vi "read_http_timeout.vi"(8 "error in (no error)":errorcluster, 11 "config_file_name":string) -> (0 "error out":errorcluster, 2 "values":cluster{"get_timeout":i32, "post_timeout":i32}, 3 "config_file_name_out":string)   [LabVIEW 2015]
uses:
  <vilib>/Utility/config.llb/Read Key (String).vi
  <vilib>/Utility/config.llb/NI_LVConfig.lvlib
panel:
  # "Devuelve datos de la sección TIMEOUT del archivo de configuración"
  # "in miliseconds"
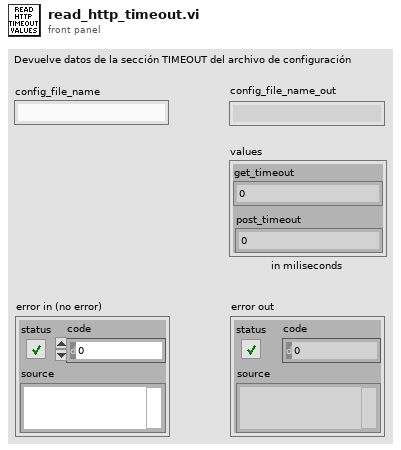
[diagram p1: front panel]
types:
  T1 = typedef "NI_LVConfig.lvlib/Config Data RefNum.ctl" = refnum<k1>
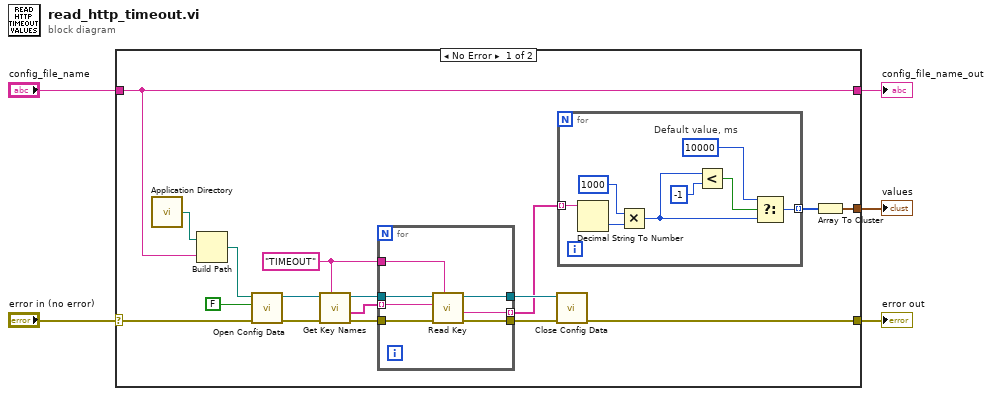
[diagram p0: block diagram]
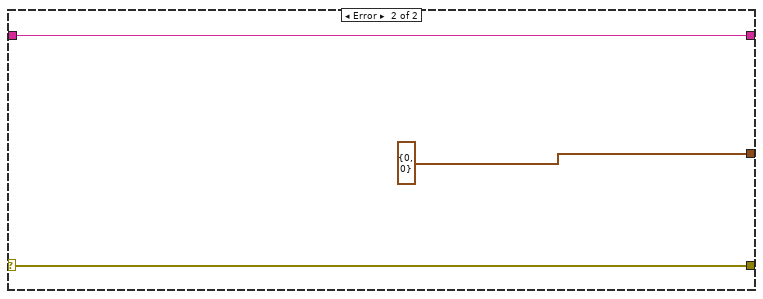
[diagram p2: hidden frame]
diagram:
  n1 = case shown="No Error" "error in (no error)" {
    selector: "error in (no error)" -> [w13 w40]
    tunnel: [w12 w40] -> w5
    tunnel: [w11 w39] -> w3
    tunnel: "config_file_name" -> [w11 w39]
    tunnel: [w8 cluster{"[0]":i32, "[1]":i32} {"[0]"=0, "[1]"=0}] -> w1
    frame No Error {
      w18 = "TIMEOUT" ("section")
      n2 = call <vilib>:"Application Directory.vi"() -> ("Application Directory"=w20:path)
      n3 = Build Path(base path=w20, name or relative path=w11) -> (appended path=w19:path)
      n4 = call <vilib>:"Open Config Data.vi"("error in (no error)"=w13, "create file if necessary (T)"=FALSE, "configuration file path"=w19) -> ("error out"=w22:errorcluster, "refnum"=w21:T1)  [unwired: 6 in, 1 out]
      n5 = call <vilib>:"Get Key Names.vi"("section"=w18, "error in (no error)"=w22, "refnum"=w21) -> ("error out"=w16:errorcluster, "key names"=w10:string[], "refnum out"=w17:T1)  [unwired: 5 in, 1 out]
      n6 = for {
        tunnel: w10 -> [w37] mode=indexing
        tunnel: [w36] -> w7 mode=indexing
        tunnel: w18 -> [w35]
        tunnel: w17 -> [w34]
        tunnel: w16 -> [w33]
        tunnel: [w32] -> w15
        tunnel: [w31] -> w14
        n7 = call-poly <vilib>:"Read Key.vi"("section"=w35, "error in (no error)"=w33, "key"=w37, "refnum"=w34) -> ("error out"=w31:errorcluster, "value"=w36:string, "refnum out"=w32:T1)  [unwired: 4 in, 1 out]
      }
      n8 = call <vilib>:"Close Config Data.vi"("error in (no error)"=w14, "refnum"=w15) -> ("error out"=w12:errorcluster)  [unwired: 8 in, 1 out]
      n9 = for {
        tunnel: w7 -> [w30] mode=indexing
        tunnel: [w27] -> w6 mode=indexing
        # "Default value, ms"
        n10 = Decimal String To Number(string=w30) -> (number=w29:i32)  [unwired: 2 in, 1 out]
        n11 = Multiply(x=1000, y=w29) -> (x*y=w23:i32)
        n12 = Less?(x=w23, y=-1) -> (x < y?=w24:bool)
        n13 = Select(t=10000, s=w24, f=w23) -> (s? t:f=w27:i32)
      }
      n14 = Array To Cluster(array=w6) -> (cluster=w8:cluster{"[0]":i32, "[1]":i32})
    }
    frame Error {
    }
  }
  "error out" <- w5
  "config_file_name_out" <- w3
  "values" <- w1
